vi "WILT Valve Test.vi"(0 "Water Valves Cluster":T8, 1 "Test Type":T7=enum."Full Valve Control", 2 "Operation Type":T11=enum."Operate As Stand-Alone EXE", 3 "Valve ON Time":dbl=100.0, 5 "Start Buttons Cluster":T9, 7 "Station Test State In":T5, 9 "Station Number":i32, 11 "Error In":errorcluster, 12 "Injection Times":T4, 13 "Day/Night Cycle":T10) -> (4 "Valve Actuation Complete":bool, 6 "Test Station Out":T5, 15 "Error Out":errorcluster)   [LabVIEW 2016] (continued)
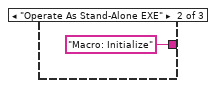
[diagram p2: hidden frame]
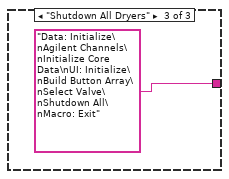
[diagram p3: hidden frame]
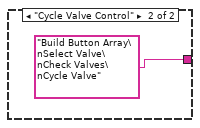
[diagram p4: hidden frame]
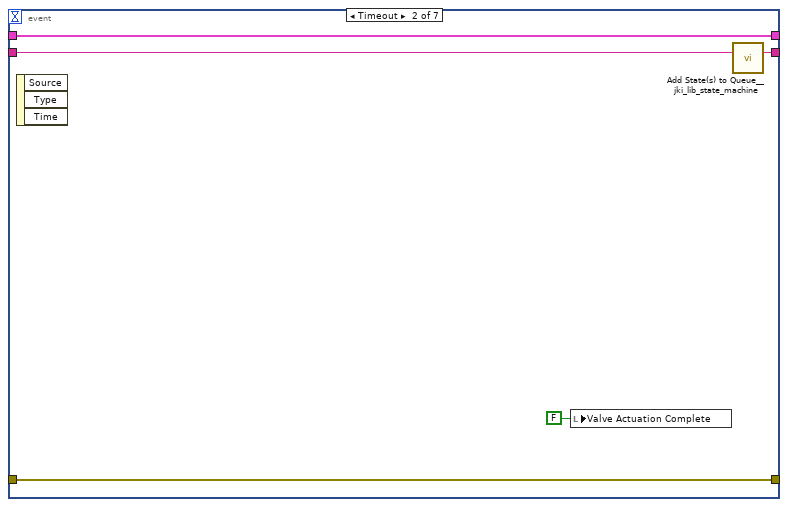
[diagram p5: hidden frame]
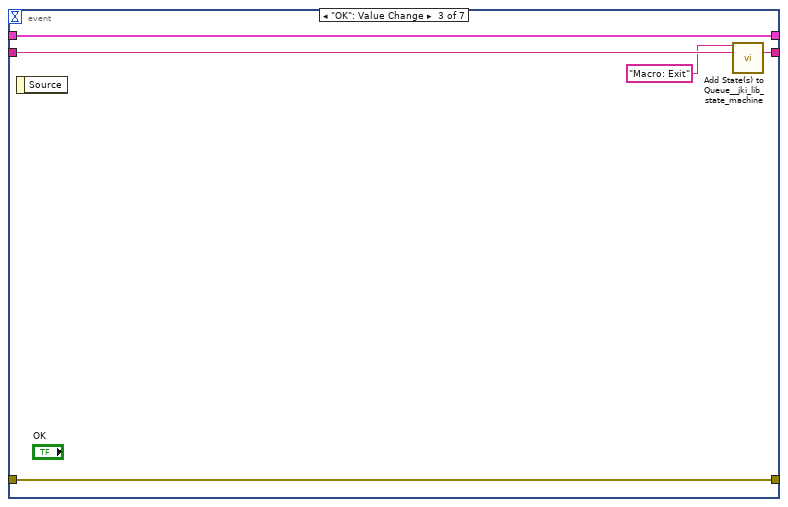
[diagram p6: hidden frame]
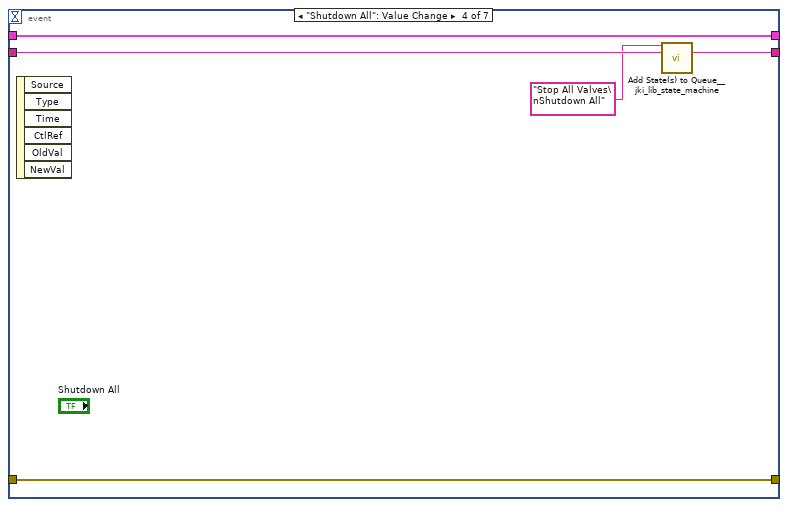
[diagram p7: hidden frame]
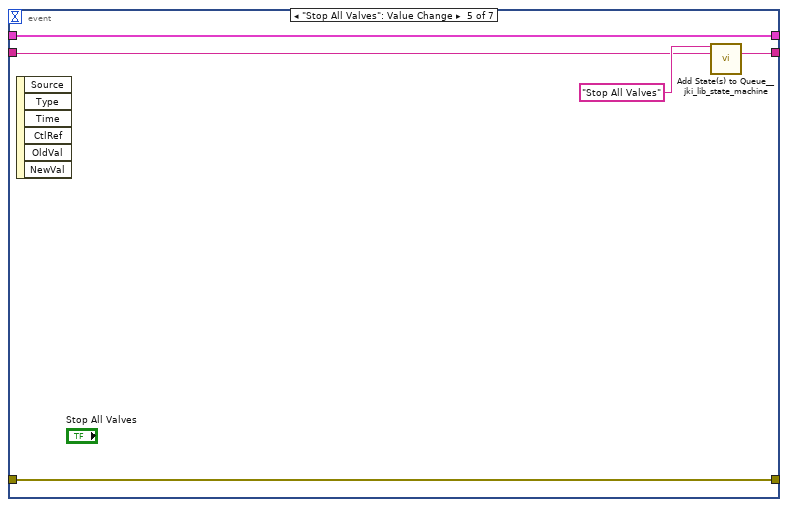
[diagram p8: hidden frame]
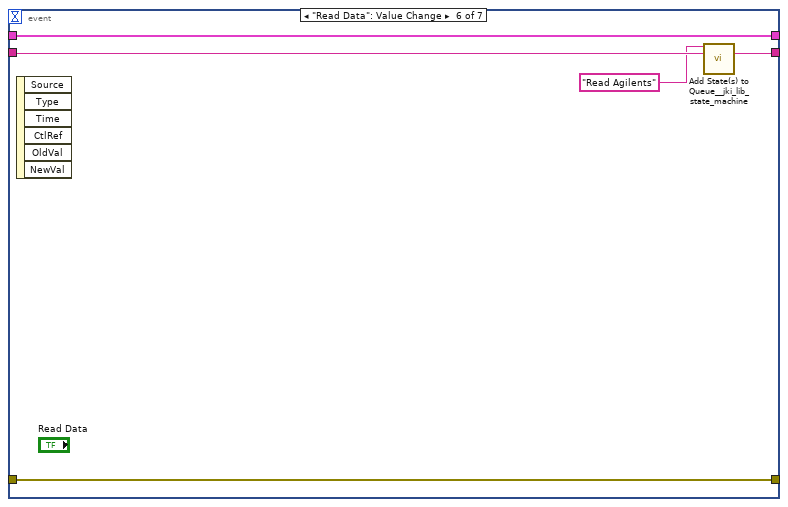
[diagram p9: hidden frame]
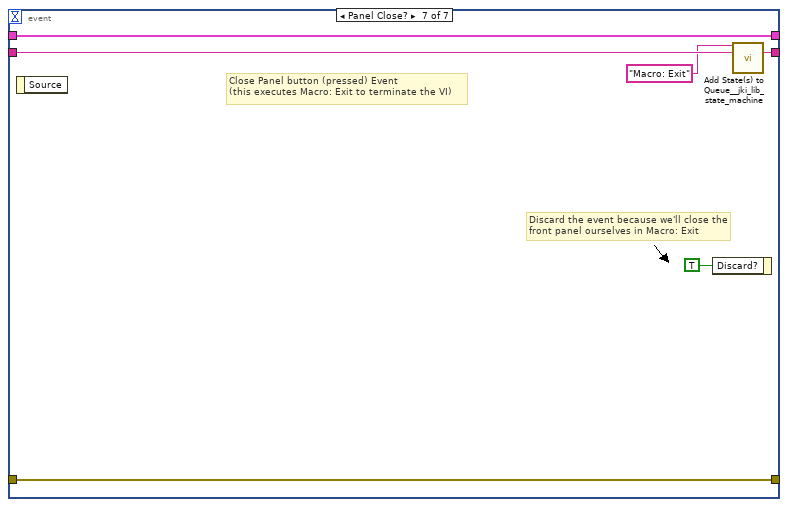
[diagram p10: hidden frame]
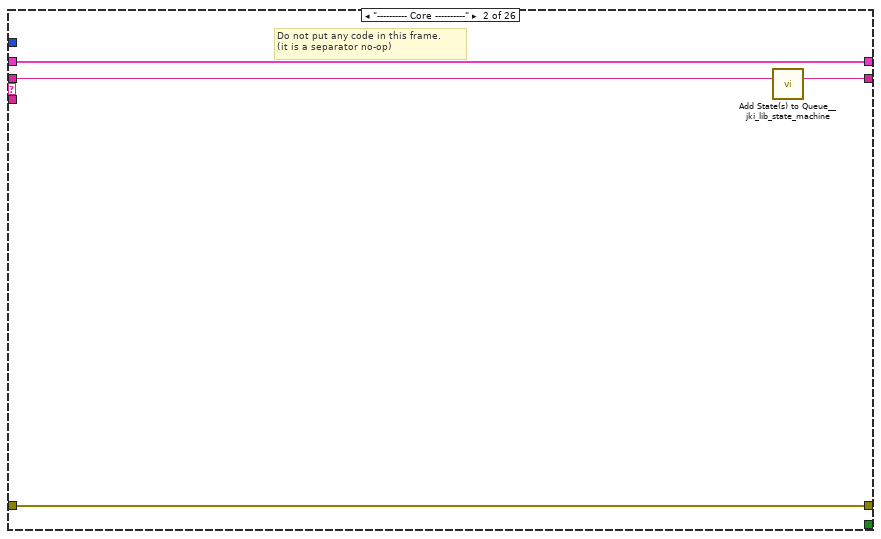
[diagram p11: hidden frame]
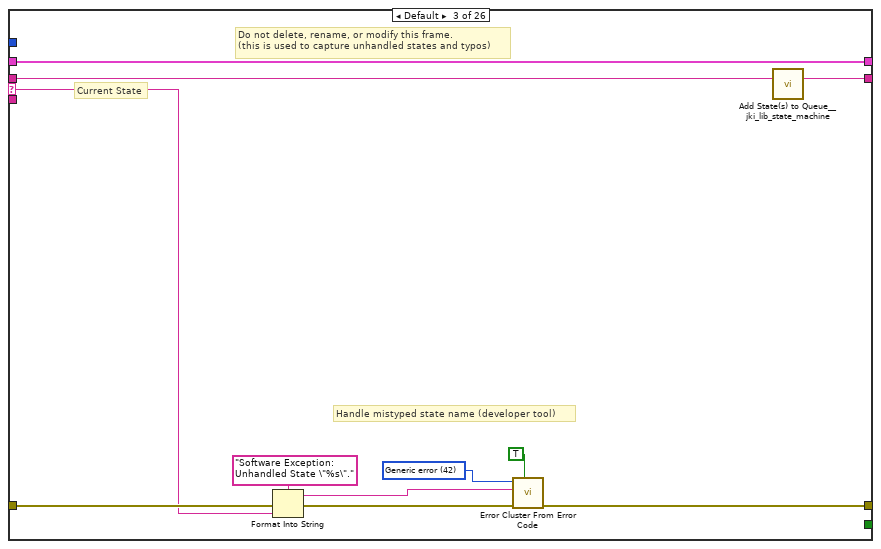
[diagram p12: hidden frame]
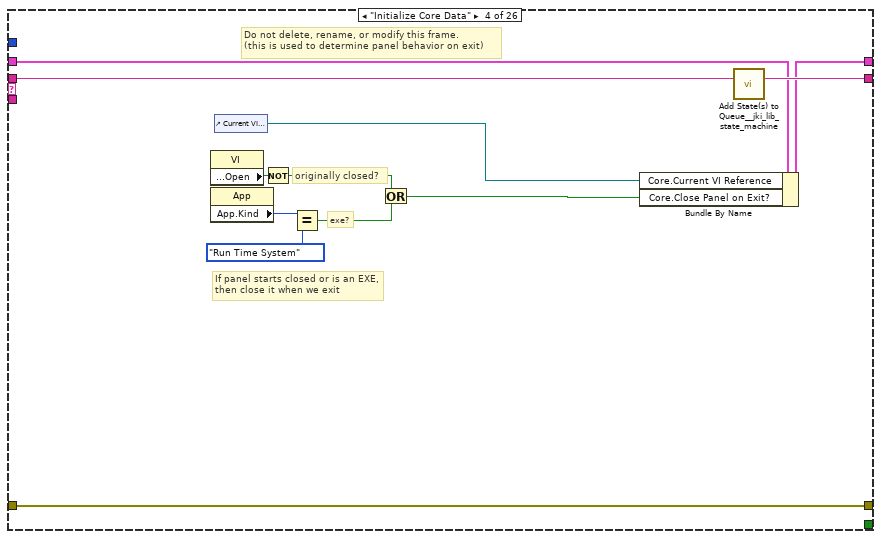
[diagram p13: hidden frame]
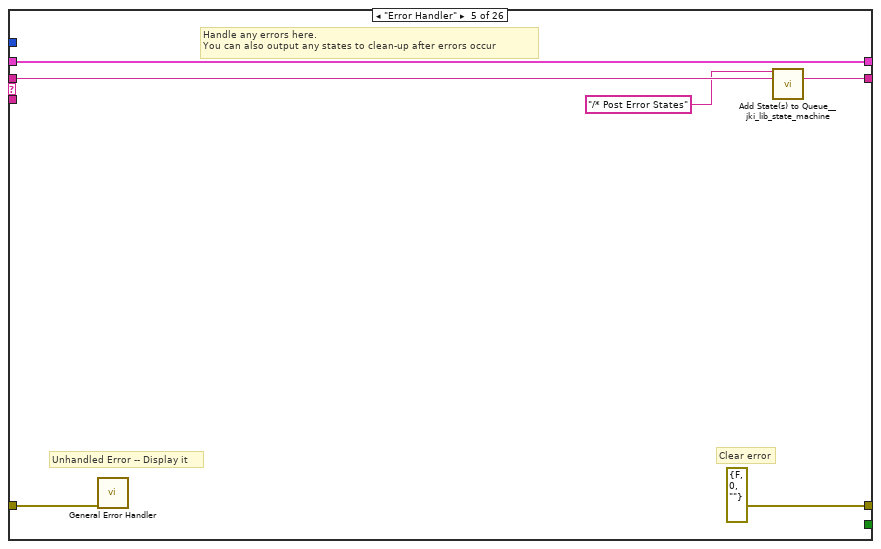
[diagram p14: hidden frame]
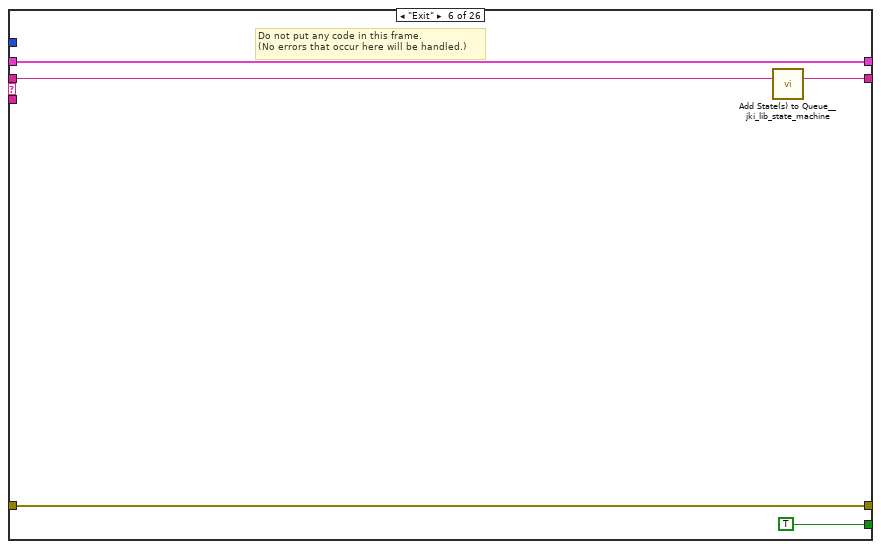
[diagram p15: hidden frame]
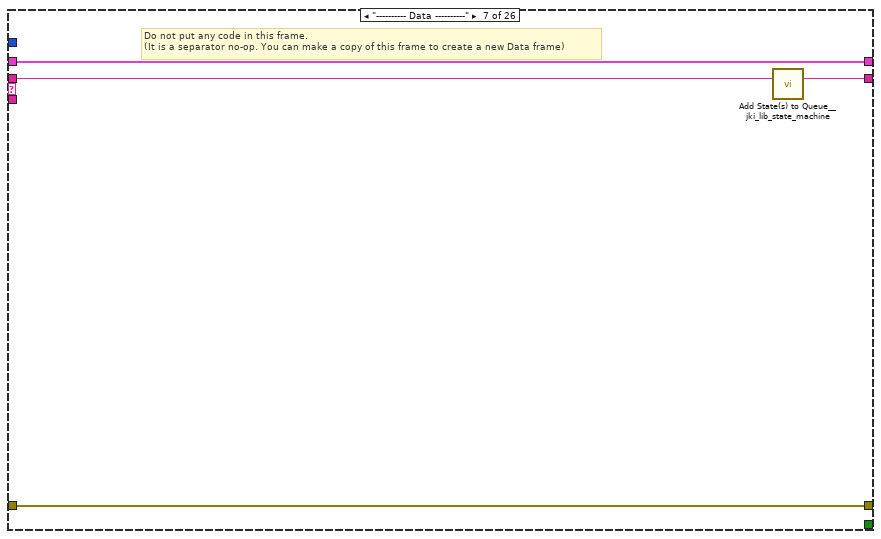
[diagram p16: hidden frame]
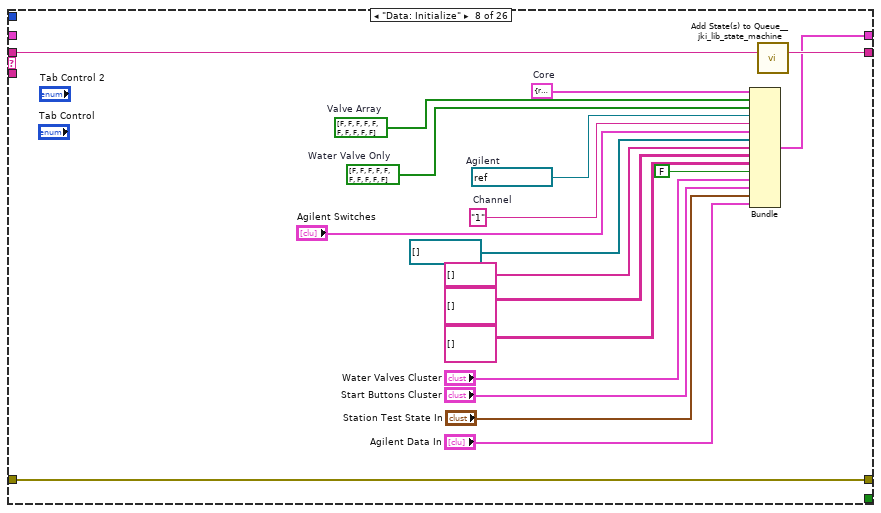
[diagram p17: hidden frame]
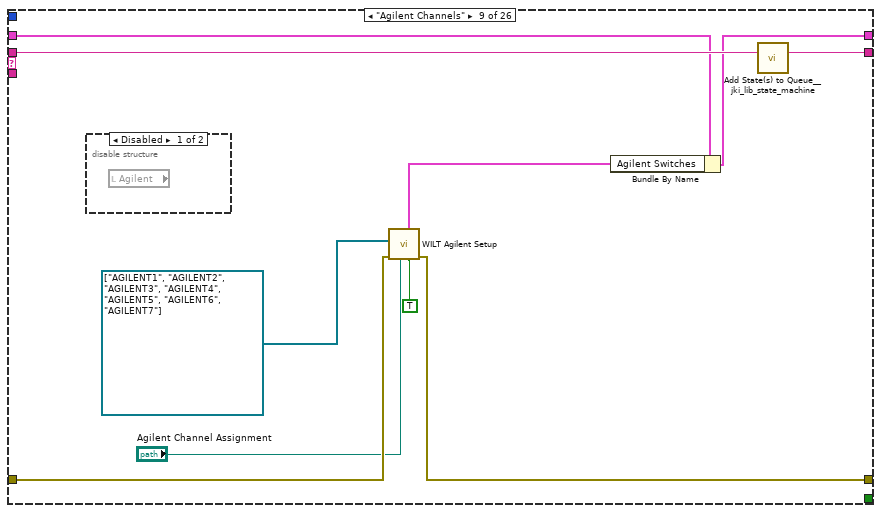
[diagram p18: hidden frame]
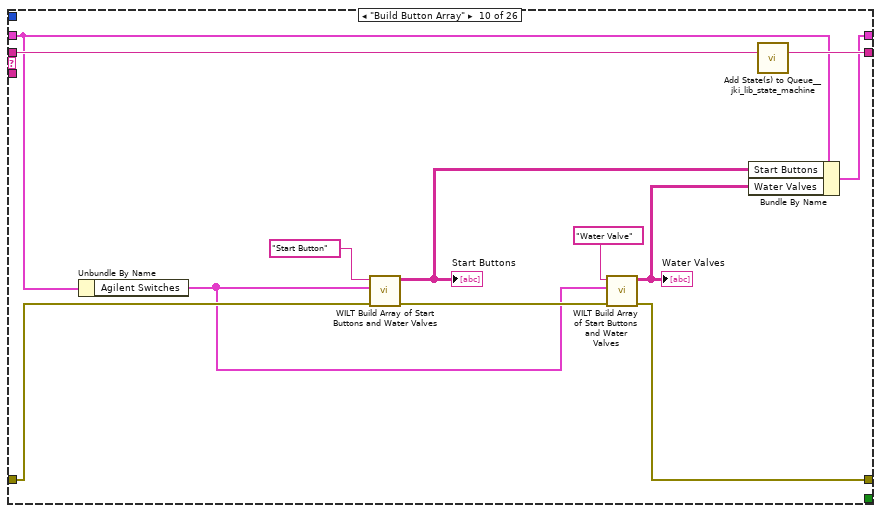
[diagram p20: hidden frame]
        n500 = call "WILT Agilent Ref Type Conversion.vi"("Agilent Ref"=w1614) -> ("VISA resource name"=w1610:refnum<visa-resource-name>)  [unwired: 14 in]
        n501 = Bundle By Name(cluster=w1612, "Agilent"=w1610, "Channel"=w1602, "Valve Act Complete"=FALSE) -> (w1611:T14)
        n502 = call <vilib>:"Add State(s) to Queue__jki_lib_state_machine.vi"("State(s) in (\"\")"=w1617) -> ("States Out"=w1616:string)  [unwired: 14 in]
      }
      frame "Check Valves" {
        n503 = Unbundle By Name(w1631) -> ("Water Valve Only"=w1625:bool[])
        n504 = Boolean To (0,1)(Boolean=w1625) -> (0, 1=w1630:i16[])
        n505 = Add Array Elements(numeric array=w1630) -> (sum=w1626:i16)
        n506 = Multiply(x=w1626, y="Current Per Valve") -> (x*y=w1628:dbl)
        n507 = Greater?(x=w1628, y="Current Limit") -> (0:w1623:bool)
        n508 = case shown="True" w1623 {
          tunnel: ["" "The Maximum Number of Valves Has Been Reached!"] -> w1624
          frame False {
          }
          frame True {
            n509 = One Button Dialog(message="Max Current \nReached. No More Valves.") -> ()  [unwired: 1 in, 1 out]
          }
        }
        "Message" <- w1624
        n510 = call <vilib>:"Add State(s) to Queue__jki_lib_state_machine.vi"("State(s) in (\"\")"=w1634) -> ("States Out"=w1633:string)  [unwired: 14 in]
      }
      frame "Cycle Valve" {
        # "Reset all of the valve controls back to OFF"
        n511 = Unbundle By Name(w1646) -> ("Agilent"=w1653:refnum<visa-resource-name>, "Channel"=w1651:string, "Station Test State In"=w1643:T5)
        n512 = case shown="\"Night Cycle\"" "Day/Night Cycle" {
          tunnel: [TRUE w1662] -> w1638
          frame "Day Cycle", Default {
          }
          frame "Night Cycle" {
            w1657 = T16 0 items=["both", "start of string", "end of string"] ("location (both)")
            n513 = call <vilib>:"Trim Whitespace.vi"("string"="Start Button" ("x"), "location (both)"=w1657) -> ("trimmed string"=w1658:string)
            n514 = local read "Label"() -> (w1661:string)
            n515 = Equal?(x=w1658, y=w1661) -> (x = y?=w1660:bool)
            n516 = case shown="True" w1660 {
              tunnel: [FALSE TRUE] -> w1662
              frame False {
              }
              frame True {
              }
            }
          }
        }
        n517 = call "UTILITY Delay mS.vi"("Error In"=w1650, "milliseconds to wait"="Delay Before Valve ON") -> ("Error Out"=w1649:errorcluster)  [unwired: 13 in]
        n518 = local read "Station Number"() -> (w1642:i32)
        n519 = case shown="True" w1638 {
          tunnel: w1653 -> [_ w1674]
          tunnel: [w1665 w1672] -> w1652
          tunnel: w1651 -> [_ w1671]
          tunnel: w1649 -> [w1665 w1670]
          tunnel: w1643 -> [_ w1669]
          tunnel: w1642 -> [_ w1668]
          tunnel: "Number of ON/OFF Cycles" -> [_ w1667]
          tunnel: "Injection Times" -> [_ w1666]
          frame False {
          }
          frame True {
            n520 = for {
              N: w1667 -> [_]
              tunnel: w1674 -> [w1687]
              tunnel: FALSE ("Set/Check (F:Set)") -> [w1686]
              shift-right: [w1681] -> w1672
              shift-left: w1670 -> [w1684]
              tunnel: w1671 -> [w1683]
              tunnel: w1669 -> [w1680]
              tunnel: w1668 -> [w1677]
              tunnel: w1666 -> [w1676]
              n521 = local read "Operation Type"() -> (w1678:T11)
              n522 = call "Switch.vi"("Channel List(empty)"=w1683, "error in (no error)"=w1684, "Open/Close (F:Close)"=w1686, "VISA Resource Name"=w1687) -> ("error out"=w1689:errorcluster, "VISA Resource Name Out"=w1688:refnum<visa-resource-name>)  [unwired: 5 in, 1 out]
              n523 = call "WILT Start Stop Timer Set.vi"("Station Number"=w1677, "Injection Times"=w1676, "Operation Type"=w1678, "Inlet Timer"="Valve ON Time", "Station Test State In"=w1680) -> ("Outlet Timer"=w1675:dbl)  [unwired: 6 in]
              n524 = call "UTILITY Delay mS.vi"("Error In"=w1689, "milliseconds to wait"=w1675) -> ("Error Out"=w1685:errorcluster)  [unwired: 13 in]
              n525 = Not(x=w1686) -> (.not. x?=w1690:bool)
              n526 = call "Switch.vi"("Channel List(empty)"=w1683, "error in (no error)"=w1685, "Open/Close (F:Close)"=w1690, "VISA Resource Name"=w1688) -> ("error out"=w1682:errorcluster)  [unwired: 5 in, 2 out]
              n527 = call "UTILITY Delay mS.vi"("Error In"=w1682, "milliseconds to wait"=w1675) -> ("Error Out"=w1681:errorcluster)  [unwired: 13 in]
            }
          }
        }
        n528 = call "WILT Update State.vi"("Station Number"=w1642, "Station Test State In in"=w1643) -> ("Station Test State In out"=w1644:T5)  [unwired: 9 in]
        n529 = flat-sequence {
          tunnel: w1652 -> [w1697]
          tunnel: [w1697] -> w1647
          tunnel: w1646 -> [w1694]
          tunnel: [w1693] -> w1645
          tunnel: w1644 -> [w1691]
          frame #0 {
            w1692 = TRUE ("Valve Act Complete")
            n530 = local write "Valve Actuation Complete"(w1692) -> ()
            n531 = Bundle By Name(cluster=w1694, "Valve Act Complete"=w1692, "Station Test State In"=w1691) -> (w1693:T14)
            n532 = local write "Start Buttons Cluster"(T9 {"Start Button 21"=FALSE, "Start Button 22"=FALSE, "Start Button 23"=FALSE, "Start Button 24"=FALSE, "Start Button 25"=FALSE, "Start Button 26"=FALSE, "Start Button 27"=FALSE, "Start Button 28"=FALSE, "Start Button 29"=FALSE, "Start Button 30"=FALSE, "Start Button 31"=FALSE, "Start Button 32"=FALSE, "Start Button 33"=FALSE, "Start Button 34"=FALSE, "Start Button 35"=FALSE, "Start Button 36"=FALSE, "Start Button 37"=FALSE, "Start Button 38"=FALSE, "Start Button 39"=FALSE, "Start Button 40"=FALSE, "Start Button 41"=FALSE, "Start Button 42"=FALSE, "Start Button 43"=FALSE, "Start Button 44"=FALSE, "Start Button 12"=FALSE, "Start Button 11"=FALSE, "Start Button 10"=FALSE, "Start Button 9"=FALSE, "Start Button 8"=FALSE, "Start Button 7"=FALSE, "Start Button 6"=FALSE, "Start Button 5"=FALSE, "Start Button 4"=FALSE, "Start Button 3"=FALSE, "Start Button 2"=FALSE, "Start Button 1"=FALSE, "Start Button 20"=FALSE, "Start Button 19"=FALSE, "Start Button 18"=FALSE, "Start Button 17"=FALSE, "Start Button 16"=FALSE, "Start Button 15"=FALSE, "Start Button 14"=FALSE, "Start Button 13"=FALSE, "Start Button 45"=FALSE, "Start Button 46"=FALSE, "Start Button 47"=FALSE, "Start Button 48"=FALSE, "Start Button 49"=FALSE, "Start Button 50"=FALSE, "Start Button 51"=FALSE, "Start Button 52"=FALSE, "Start Button 53"=FALSE, "Start Button 54"=FALSE, "Start Button 55"=FALSE, "Start Button 56"=FALSE} ("Start Buttons Cluster")) -> ()
            n533 = local write "Water Valves Cluster"(T8 {"Valve 1"=FALSE, "Valve 2"=FALSE, "Valve 3"=FALSE, "Valve 4"=FALSE, "Valve 5"=FALSE, "Valve 6"=FALSE, "Valve 7"=FALSE, "Valve 8"=FALSE, "Valve 9"=FALSE, "Valve 10"=FALSE, "Valve 11"=FALSE, "Valve 12"=FALSE, "Valve 13"=FALSE, "Valve 14"=FALSE, "Valve 15"=FALSE, "Valve 16"=FALSE, "Valve 17"=FALSE, "Valve 18"=FALSE, "Valve 19"=FALSE, "Valve 20"=FALSE, "Valve 21"=FALSE, "Valve 22"=FALSE, "Valve 23"=FALSE, "Valve 24"=FALSE, "Valve 25"=FALSE, "Valve 26"=FALSE, "Valve 27"=FALSE, "Valve 28"=FALSE, "Valve 29"=FALSE, "Valve 30"=FALSE, "Valve 31"=FALSE, "Valve 32"=FALSE, "Valve 33"=FALSE, "Valve 34"=FALSE, "Valve 35"=FALSE, "Valve 36"=FALSE, "Valve 37"=FALSE, "Valve 38"=FALSE, "Valve 39"=FALSE, "Valve 40"=FALSE, "Valve 41"=FALSE, "Valve 42"=FALSE, "Valve 43"=FALSE, "Valve 44"=FALSE, "Valve 45"=FALSE, "Valve 46"=FALSE, "Valve 47"=FALSE, "Valve 48"=FALSE, "Valve 49"=FALSE, "Valve 50"=FALSE, "Valve 51"=FALSE, "Valve 52"=FALSE, "Valve 53"=FALSE, "Valve 54"=FALSE, "Valve 55"=FALSE, "Valve 56"=FALSE} ("Water Valves Cluster")) -> ()
          }
        }
        n534 = call <vilib>:"Add State(s) to Queue__jki_lib_state_machine.vi"("State(s) in (\"\")"=w1655) -> ("States Out"=w1654:string)  [unwired: 14 in]
      }
      frame "Control Valve" {
        n535 = Unbundle By Name(w1704) -> ("Agilent"=w1701:refnum<visa-resource-name>, "Channel"=w1700:string)
        n536 = call "Agilent 34970 Set Switch.vi"("error in (no error)"=w1702, "Channel"=w1700, "VISA Refnum in"=w1701) -> ("error out"=w1703:errorcluster, "Success"=→"Success":bool, "VISA Resource Name Out"=→"Channel State?":refnum<visa-resource-name>)  [unwired: 5 in, 1 out]
        n537 = call <vilib>:"Add State(s) to Queue__jki_lib_state_machine.vi"("State(s) in (\"\")"=w1706) -> ("States Out"=w1705:string)  [unwired: 14 in]
      }
      frame "Shutdown All" {
        n538 = Unbundle By Name(w1715) -> ("Start Buttons"=w1710:string[][])
        n539 = Index Array(array=w1710, index (col) #1=2 ("disabled index (col)"), index (col) #2=1 ("disabled index (col)")) -> (element #1=w1711:string[], element #2=w1707:string[])  [unwired: 2 in]
        n540 = for {
          tunnel: w1711 -> [w1722] mode=indexing
          tunnel: [w1719] -> w1709 mode=indexing
          tunnel: [FALSE] -> w1708 mode=indexing
          n541 = Decimal String To Number(string=w1722, default (0L)=u8 0 ("default (0 I32)")) -> (number=w1721:u8)  [unwired: 1 in, 1 out]
          n542 = call "WILT Agilent Ref Type Conversion.vi"("Agilent Ref"=w1721) -> ("VISA resource name"=w1719:refnum<visa-resource-name>)  [unwired: 14 in]
        }
        n543 = for {
          tunnel: w1709 -> [w1730] mode=indexing
          tunnel: w1708 -> [w1729] mode=indexing
          shift-right: [w1724] -> _
          shift-left: _ -> [w1727]
          tunnel: w1707 -> [w1726] mode=indexing
          w1723 = 100.0  # ON Time
          n544 = call "Switch.vi"("Channel List(empty)"=w1726, "error in (no error)"=w1727, "Open/Close (F:Close)"=w1729, "VISA Resource Name"=w1730) -> ("error out"=w1732:errorcluster, "VISA Resource Name Out"=w1731:refnum<visa-resource-name>)  [unwired: 5 in, 1 out]
          n545 = call "UTILITY Delay mS.vi"("Error In"=w1732, "milliseconds to wait"=w1723) -> ("Error Out"=w1728:errorcluster)  [unwired: 13 in]
          n546 = Not(x=w1729) -> (.not. x?=w1733:bool)
          n547 = call "Switch.vi"("Channel List(empty)"=w1726, "error in (no error)"=w1728, "Open/Close (F:Close)"=w1733, "VISA Resource Name"=w1731) -> ("error out"=w1725:errorcluster)  [unwired: 5 in, 2 out]
          n548 = call "UTILITY Delay mS.vi"("Error In"=w1725, "milliseconds to wait"=w1723) -> ("Error Out"=w1724:errorcluster)  [unwired: 13 in]
        }
        n549 = call <vilib>:"Add State(s) to Queue__jki_lib_state_machine.vi"("State(s) in (\"\")"=w1717) -> ("States Out"=w1716:string)  [unwired: 14 in]
      }
      frame "Stop All Valves" {
        # "Shutdown all valves"
        n550 = Unbundle By Name(w1735) -> ("Agilent Switches"=w1734:T2[])
        n551 = for {
          N: 56 -> [_]
          shift-right: [w1745] -> w1736
          shift-left: w1737 -> [w1746]
          tunnel: w1734 -> [w1741]
          i -> [w1743]
          n552 = Increment(x=w1743) -> (x+1=w1742:i32)
          n553 = call "WILT Turn Valve Off.vi"("Remote Station"=FALSE, "Error In"=w1746, "Station Index"=w1742, "Agilent Valve and Switch Locations"=w1741) -> ("Error Out"=w1745:errorcluster)  [unwired: 7 in]
        }
        n554 = call <vilib>:"Add State(s) to Queue__jki_lib_state_machine.vi"("State(s) in (\"\")"=w1740) -> ("States Out"=w1739:string)  [unwired: 14 in]
      }
      frame "Read Agilents" {
        n555 = Unbundle By Name(w1749) -> ("Agilent Data In"=w1748:T1)
        n556 = call "WILT Agilent Read 5 Units.vi"("Agilent Refs"=refnum<visa-resource-name>[] ["AGILENT1", "AGILENT2", "AGILENT3", "AGILENT4", "AGILENT5", "AGILENT6", "AGILENT7"], "Data Array"=w1748) -> ("Data Out Array"=→"Agilent Data Out":T1)  [unwired: 14 in, 3 out]
        n557 = call <vilib>:"Add State(s) to Queue__jki_lib_state_machine.vi"("State(s) in (\"\")"=w1753) -> ("States Out"=w1752:string)  [unwired: 14 in]
      }
    }
  }
  "Error Out" <- w5
  n558 = Unbundle By Name(w3) -> ("Valve Act Complete"=→"Valve Actuation Complete":bool, "Station Test State In"=→"Test Station Out":T5)
